vi "Draw Exponential Decay.vi"(1 "time":dbl[](array[numeric]), 2 "B":dbl, 3 "A":dbl, 4 "tau":dbl) -> (0 "ExponentialOut":dbl[](array[numeric]))   [LabVIEW 2014, in "Math Utilities.lvlib"]
doc: "Draw an exponential decay given the time constant, scale and offset for a defined time interval."
uses:
  Math Utilities.lvlib
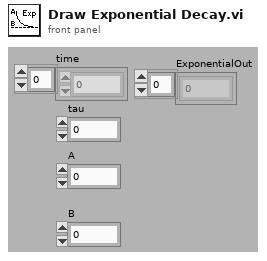
[diagram p1: front panel]
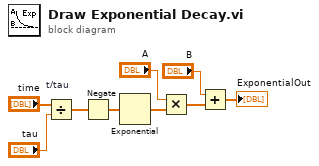
[diagram p0: block diagram]
diagram:
  n1 = Divide "t/tau"(x="time", y="tau") -> (x/y=w6:dbl[])
  n2 = Negate(x=w6) -> (-x=w7:dbl[])
  n3 = Exponential(1:w7) -> (0:w1:dbl[])
  n4 = Multiply(x="A", y=w1) -> (x*y=w3:dbl[])
  n5 = Add(x="B", y=w3) -> (x+y=→"ExponentialOut":dbl[])
